vi "MSScript_Calc_ArraySeries.vi"(6 "Value Error?":bool[](array[boolean]), 8 "ArrayVariable in":ext[](array[numeric]), 9 "Param Items":i32) -> (0 "ArrayVariable out":ext[](array[numeric]), 2 "CmdError?":bool)   [LabVIEW 2018, in "MSScript.lvclass"]
uses:
  MSScript.lvclass
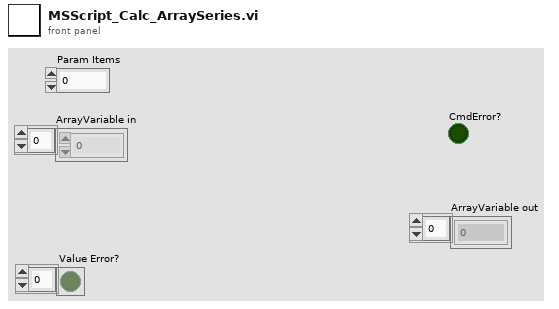
[diagram p1: front panel]
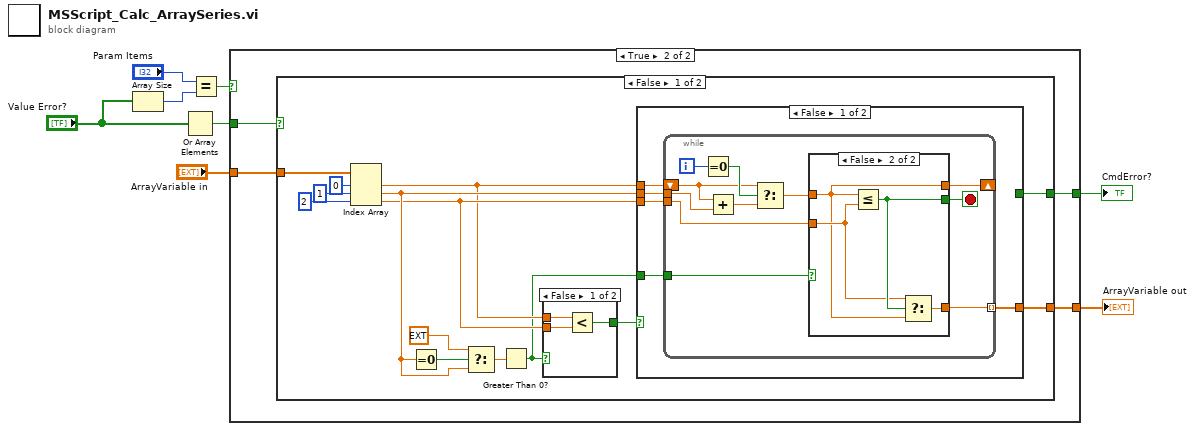
[diagram p0: block diagram]
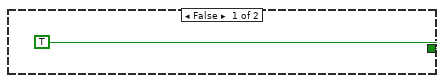
[diagram p2: hidden frame]
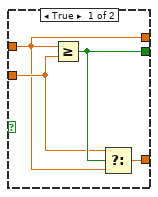
[diagram p3: hidden frame]
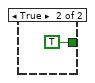
[diagram p4: hidden frame]
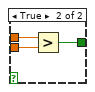
[diagram p5: hidden frame]
diagram:
  n1 = Array Size(array="Value Error?") -> (size(s)=w5:i32)
  n2 = Or Array Elements(Boolean array="Value Error?") -> (logical OR=w7:bool)
  n3 = Equal?(x="Param Items", y=w5) -> (x = y?=w3:bool)
  n4 = case shown="True" w3 {
    tunnel: [TRUE w10] -> w2
    tunnel: w7 -> [_ w13]
    tunnel: [_ w11] -> w8
    tunnel: "ArrayVariable in" -> [_ w12]
    frame False {
    }
    frame True {
      n5 = case shown="False" w13 {
        tunnel: w12 -> [w27 _]
        tunnel: [w15 _] -> w11
        tunnel: [w16 _] -> w10
        frame False {
          n6 = Index Array(array=w27, index #1=0 ("index"), index #2=1 ("index"), index #3=2 ("index")) -> (element #1=w17:ext, element #2=w19:ext, element #3=w18:ext)
          n7 = Equal To 0?(x=w19) -> (x = 0?=w23:bool)
          n8 = Select(t=ext 1.0, s=w23, f=w19) -> (s? t:f=w21:ext)
          n9 = Greater Than 0?(x=w21) -> (x > 0?=w14:bool)
          n10 = case shown="False" w14 {
            tunnel: w17 -> [w55 w58]
            tunnel: w18 -> [w54 w57]
            tunnel: [w53 w56] -> w20
            frame False {
              n11 = Less?(x=w55, y=w54) -> (x < y?=w53:bool)
            }
            frame True {
              n12 = Greater?(x=w58, y=w57) -> (0:w56:bool)
            }
          }
          n13 = case shown="False" w20 {
            tunnel: w19 -> [w32 _]
            tunnel: w18 -> [w30 _]
            tunnel: w17 -> [w31 _]
            tunnel: [_ TRUE] -> w16
            tunnel: [w29 _] -> w15
            tunnel: w14 -> [w28 _]
            frame False {
              n14 = while {
                tunnel: w32 -> [w34]
                tunnel: w30 -> [w39]
                tunnel: [w37] -> w29 mode=indexing
                tunnel: w28 -> [w41]
                shift-right: [w33] -> _
                shift-left: w31 -> [w35]
                i -> [w43]
                stop <- w38 stop-if-true
                n15 = Equal To 0?(x=w43) -> (x = 0?=w42:bool)
                n16 = Add(x=w35, y=w34) -> (x+y=w36:ext)
                n17 = Select(t=w35, s=w42, f=w36) -> (s? t:f=w40:ext)
                n18 = case shown="False" w41 {
                  tunnel: w40 -> [w44 w48]
                  tunnel: w39 -> [w46 w50]
                  tunnel: [w47 w51] -> w38
                  tunnel: [w45 w49] -> w37
                  tunnel: [w44 w48] -> w33
                  frame True {
                    n19 = Greater Or Equal?(x=w44, y=w46) -> (x >= y?=w47:bool)
                    n20 = Select(t=w46, s=w47, f=w44) -> (s? t:f=w45:ext)
                  }
                  frame False {
                    n21 = Less Or Equal?(x=w48, y=w50) -> (x <= y?=w51:bool)
                    n22 = Select(t=w50, s=w51, f=w48) -> (s? t:f=w49:ext)
                  }
                }
              }
            }
            frame True {
            }
          }
        }
        frame True {
        }
      }
    }
  }
  "ArrayVariable out" <- w8
  "CmdError?" <- w2
